vi "Generate RP for CP CV Sweep.vi"(0 "Start":i64, 5 "Step":i64, 7 "Stop":i64, 11 "error in (no error)":errorcluster) -> (4 "RP for CP CV":i64[](array[numeric]), 15 "error out":errorcluster)   [LabVIEW 2012]
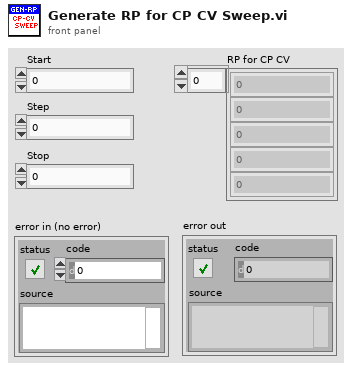
[diagram p1: front panel]
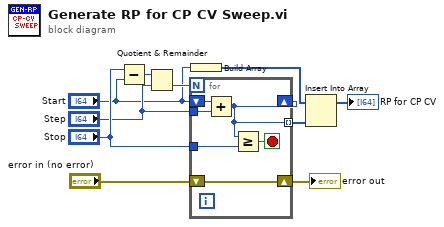
[diagram p0: block diagram]
diagram:
  n1 = Subtract(x="Stop", y="Start") -> (x-y=w9:i64)
  n2 = Quotient & Remainder(x=w9, y="Step") -> (floor(x/y)=w7:i64)  [unwired: 1 out]
  n3 = for {
    N: w7 -> [_]
    tunnel: "Stop" -> [w15]
    tunnel: "Step" -> [w16]
    shift-right: [w13] -> _
    shift-left: "Start" -> [w12]
    tunnel: [w13] -> w6 mode=indexing
    shift-right: [w11] -> w1
    shift-left: "error in (no error)" -> [w11]
    stop <- w14 stop-if-true
    n4 = Add(x=w12, y=w16) -> (x+y=w13:i64)
    n5 = Greater Or Equal?(x=w13, y=w15) -> (x >= y?=w14:bool)
  }
  "error out" <- w1
  n6 = Build Array("Start") -> (w3:i64[])
  n7 = Insert Into Array(array=w3, new element=w6) -> (→"RP for CP CV":i64[])  [unwired: 1 in]
